vi "Get Cache.vi"(11 "ConfigManagerCollection in":refnum<class "ConfigManagerCollection.lvclass">) -> (1 "found?":bool, 2 "Cache":refnum<class "ConfigManager.Cache.lvclass">, 3 "ConfigManagerCollection out":refnum<class "ConfigManagerCollection.lvclass">)   [LabVIEW 2013, in "CfgManager.lvlib" / "ConfigManagerCollection.lvclass"]
uses:
  ConfigManagerCollection.lvclass
  Cache/ConfigManager.Cache.lvclass
  ConfigManagerCollection.lvclass/ConfigManagerCollection.ctl
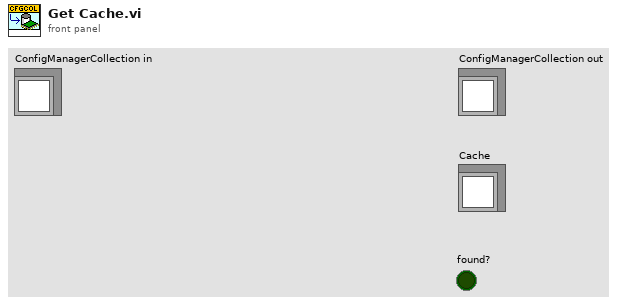
[diagram p1: front panel]
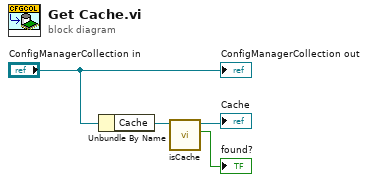
[diagram p0: block diagram]
diagram:
  n1 = Unbundle By Name("ConfigManagerCollection in") -> ("Cache"=w3:refnum<class "ConfigManager.Cache.lvclass">)
  n2 = call "isCache.vi"("ConfigManager.Cache in"=w3) -> ("isCache?"=→"found?":bool, "ConfigManager.Cache out"=→"Cache":refnum<class "ConfigManager.Cache.lvclass">)  [unwired: 9 in]
  "ConfigManagerCollection out" <- "ConfigManagerCollection in"
